vi "Navigation_no s curve may 2.vi"() -> ()   [LabVIEW 2015]
uses:
  <vilib>/myRIO/Instrument Drivers/Onboard IO/PWM/typedefs/PWM Reference.ctl
  <vilib>/myRIO/Common/Instrument Driver Framework/Utilities/typedefs/myRIO Generic Hardware Reference.ctl
  <vilib>/myRIO/Common/Instrument Driver Framework/Utilities/typedefs/Hardware Version Enum.ctl
  <vilib>/myRIO/Common/Instrument Driver Framework/Utilities/typedefs/myRIO v1.0 Reference.ctl
  <vilib>/myRIO/Common/Instrument Driver Framework/Utilities/typedefs/Generic FPGA Reference.ctl
  <vilib>/myRIO/Common/Instrument Driver Framework/myRIO v1.0/PWM/typedefs/PWM Channels Enum.ctl
  <vilib>/myRIO/Instrument Drivers/Onboard IO/PWM/typedefs/PWM Configuration.ctl
  <vilib>/userdefined/High Color/nirio_resource_hc.ctl
  <vilib>/myRIO/Common/Instrument Driver Framework/myRIO v1.0/PWM/vis/myRIO v1.1 Open PWM.vi
  <vilib>/myRIO/Common/Instrument Driver Framework/Utilities/vis/Validate Channels.vi
  <vilib>/myRIO/Common/Instrument Driver Framework/myRIO v1.0/PWM/vis/myRIO v1.0 Reserve PWM.vi
  <vilib>/myRIO/Common/Instrument Driver Framework/myRIO v1.0/PWM/vis/myRIO v1.0 Build MUX Configuration PWM.vi
  <vilib>/myRIO/Common/Instrument Driver Framework/myRIO v1.0/Resource Manager/vis/myRIO v1.0 Reserve Channel List.vi
  <vilib>/myRIO/Common/Instrument Driver Framework/myRIO v1.0/Resource Manager/vis/myRIO v1.0 Create Configuration List.vi
  <vilib>/myRIO/Common/Instrument Driver Framework/myRIO v1.0/Resource Manager/vis/myRIO v1.0 Reserve Channel.vi
  <vilib>/myRIO/Common/Instrument Driver Framework/myRIO v1.0/Resource Manager/vis/myRIO v1.0 Unreserve Channel.vi
  <vilib>/myRIO/Common/Instrument Driver Framework/myRIO v1.0/Resource Manager/vis/myRIO v1.0 Build Mutex Name.vi
  <vilib>/FPGAPlugInAG/myRIO-1900/niLvFpga_Open_myRIO-1900.vi
  <vilib>/rvi/interface/common/dynamic/niFpgaDynamicAddResources.vi
  <vilib>/myRIO/Common/Instrument Driver Framework/Utilities/vis/FPGA Ref Manager.vi
  <vilib>/Utility/error.llb/Error Cluster From Error Code.vi
  <vilib>/myRIO/Common/Instrument Driver Framework/Utilities/vis/Ref Counter.vi
  <vilib>/rvi/errors/niLvFpgaAdjustHostInterfaceError.vi
  <vilib>/Utility/VariantDataType/GetNumericInfo.vi
  <vilib>/myRIO/Common/Instrument Driver Framework/myRIO v1.0/myRIO v1.1 Open.vi
  <vilib>/myRIO/Common/Instrument Driver Framework/Utilities/vis/IO Manager.vi
  <vilib>/myRIO/Common/Instrument Driver Framework/Utilities/vis/Configuration Manager.vi
  <vilib>/myRIO/Common/Instrument Driver Framework/myRIO v1.0/Resource Manager/vis/myRIO v1.0 Configure IO.vi
  <vilib>/myRIO/Common/Instrument Driver Framework/myRIO v1.0/myRIO v1.0 Close.vi
  <vilib>/myRIO/Common/Instrument Driver Framework/myRIO v1.0/PWM/vis/myRIO v1.0 Write PWM.vi
  <vilib>/addons/control/pid/pid.llb/PID (DBL).vi
  <vilib>/rvi/interface/nirviOpenFPGA/nirviOpenFPGA.xnode
  FPGA Bitfiles/NavigationProjec_FPGATarget2_FPGAMainNavigati_PWPHW8gwDxI.lvbitx
  <vilib>/rvi/interface/nirviReadWriteControl/nirviReadWriteControl.xnode
  <vilib>/myRIO/Instrument Drivers/Onboard IO/PWM/vis/myRIO PWM Open.xnode
  <vilib>/myRIO/Instrument Drivers/Onboard IO/PWM/PWM.lvlib
  <vilib>/myRIO/Instrument Drivers/Utilities/Utilities.lvlib
  NiFpgaLv.dll
  <vilib>/rvi/interface/Simulation/niFpgaSimulationCallBeginRW.vi
  <vilib>/addons/control/pid/NI_PID_pid.lvlib
panel:
  out "xstart_return":dbl
  out "goal reached 2":bool=TRUE
  out "percent away from x goal 2":dbl
  out "forward reverse":dbl
  out "big red button":i16
  out "y1ahead":dbl
  out "angle error":dbl
  out "percent away from x goal":dbl
  out "y desired":dbl
  out "slope desired":dbl
  out "orientation theta desired":dbl
  out "current angle":dbl
  out "current y":dbl
  out "current x":dbl
  out "mining angle":dbl
  out "mining y":dbl
  out "mining x":dbl
  out "mining location":dbl=1.0
  out "distance to goal":dbl
  out "loc_y":dbl
  out "loc_x":dbl
  out "loc_theta":dbl
  in  "motor killswitch":bool=TRUE
  in  "set start position":bool
  in  "dumping complete":bool
  in  "digging complete?":bool
  in  "position good?":bool
  in  "state":dbl
  in  "x goal":dbl=9.0
  in  "Encoder Reset":bool
  out "scale":dbl=1.0
  out "reset x y 2":dbl
  out "stop motors":dbl
  out "encoder stop switch":dbl=1.0
  out "left wheels actual pwm":dbl
  out "right wheels actual pwm":dbl
  out "desired pwm right":dbl
  out "desired pwm left":dbl
  out "left setpoint":dbl
  out "right setpoint":dbl
  in  "PID Settings":enum32{"Right PID PWM", "Left PID PWM"}(tab)
  in  "output range right":cluster{"output high":dbl, "output low":dbl}={"output high"=0.13333, "output low"=-0.13333} {"output low" format="%.6f"; "output high" format="%.5f"}
  in  "PID gains right":T1={"proportional gain (Kc)"=0.002, "integral time (Ti, min)"=7e-07, "derivative time (Td, min)"=0.0} {"derivative time (Td, min)" format="%.8f"; "integral time (Ti, min)" format="%.8f"; "proportional gain (Kc)" format="%.8f"}
  out "dt out (s) right":dbl format="%.3f"
  out "PID feedback Right":dbl
  out "Elapsed Time (s) Right":dbl caption="Elapsed Time (s)"
  in  "pid reset right":bool
  in  "output range left":cluster{"output high":dbl, "output low":dbl}={"output high"=0.13333, "output low"=-0.13333} {"output low" format="%.6f"; "output high" format="%.5f"}
  in  "PID gains left":T1={"proportional gain (Kc)"=0.002, "integral time (Ti, min)"=7e-07, "derivative time (Td, min)"=0.0} {"derivative time (Td, min)" format="%.8f"; "integral time (Ti, min)" format="%.8f"; "proportional gain (Kc)" format="%.8f"}
  out "dt out (s) left":dbl format="%.3f"
  out "PID feedback Left":dbl
  out "Elapsed Time (s) Left":dbl caption="Elapsed Time (s)"
  in  "pid reset left":bool
  out "start angle":dbl=1.0
  out "start x":dbl=1.0
  out "start y":dbl
  in  "stuff that i dont want to mess with right now":T2(tab)
  out "RM Linear Velocity (rot/s)":dbl
  out "RR Rot Velocity (rot/s)":dbl
  out "LR Rot Velocity (rot/s)":dbl
  out "LM Rot Velocity (rot/s)":dbl
  out "LF Rot Velocity (rot/s)":dbl
  out "RF Linear Velocity (rot/s)":dbl
  out "Tick Count(mSec) 2":u32 caption="Tick Count(mSec)"
  out "y traveled 2":dbl
  out "x traveled 2":dbl
  out "y position 2":dbl
  out "x position 2":dbl
  out "y dot 2":dbl
  out "distance traveled 2":dbl
  out "psi dot 2":dbl
  out "x dot 2":dbl
  out ".not. x? 2":bool
  out ".not. x? 3":bool
  out "goal reached":bool=TRUE
  out "avg ENC.B":dbl
  out "avg ENC.A":dbl
  out "ENC.B_c.CNTR":i32
  out "ENC.B_b.CNTR":i32
  out "ENC.B_a.CNTR":i32
  out "ENC.A_c.CNTR":i32
  out "ENC.A_b.CNTR":i32
  out "ENC.A_a.CNTR":i32
  out "stage set point parameters":T3(tab)
  in  "x straight 1 end":dbl=2.0
  in  "ypstart straight 1":dbl
  in  "ystart":dbl=1.0
  in  "yend straight 1":dbl=2.0
  in  "ypend straight 1":dbl
  out "a":dbl
  out "b":dbl
  out "c":dbl
  out "d":dbl
  out "x turn end":dbl=7.0
  out "x straight 2 end":dbl=10.0
  in  "mining y 1":dbl=2.0
  in  "mining angle 1":dbl
  in  "mining x 1":dbl=9.0
  in  "mining angle -1":dbl
  in  "mining y -1":dbl=4.0
  in  "mining x -1":dbl=9.0
  out "left pwm":dbl(graph)
  out "right pwm":dbl(graph)
  out "SYS.SELECTA":u8 format="%08b"
  in  "R Min Linear Velocity (ft/s)":dbl=-2.0 format="%#_13g"
  in  "R Max Linear Velocity (ft/s)":dbl=2.0 format="%#_13g"
  in  "L Min Linear Velocity (ft/s)":dbl=-2.0 format="%#_13g"
  in  "L Max Linear Velocity (ft/s)":dbl=2.0 format="%#_13g"
  out "Current Rot Velocity (rot/s)":T4(graph)
  # "Position Information"
  # "move cases along"
  # "end state 0\ngo to state 1"
  # "end state 1\ngo to state 2"
  # "end state 2\ngo to state 3"
  # "end state 3\ngo to state 4"
  # "end state 4\ngo to state 0"
  # "same thing, redundant \nbut can be changed to \nsomething useful later"
  # "this must be true to \ninitialize the routine"
  # "go through the 3\n movement cases"
  # "go through the 3\n movement cases"
  # "Stop Flags \n1=go \n0=stop"
  # "PWM Setpoint"
  # "Initial condtions"
  # "Encoder Values"
  # "Motor Control Parameters"
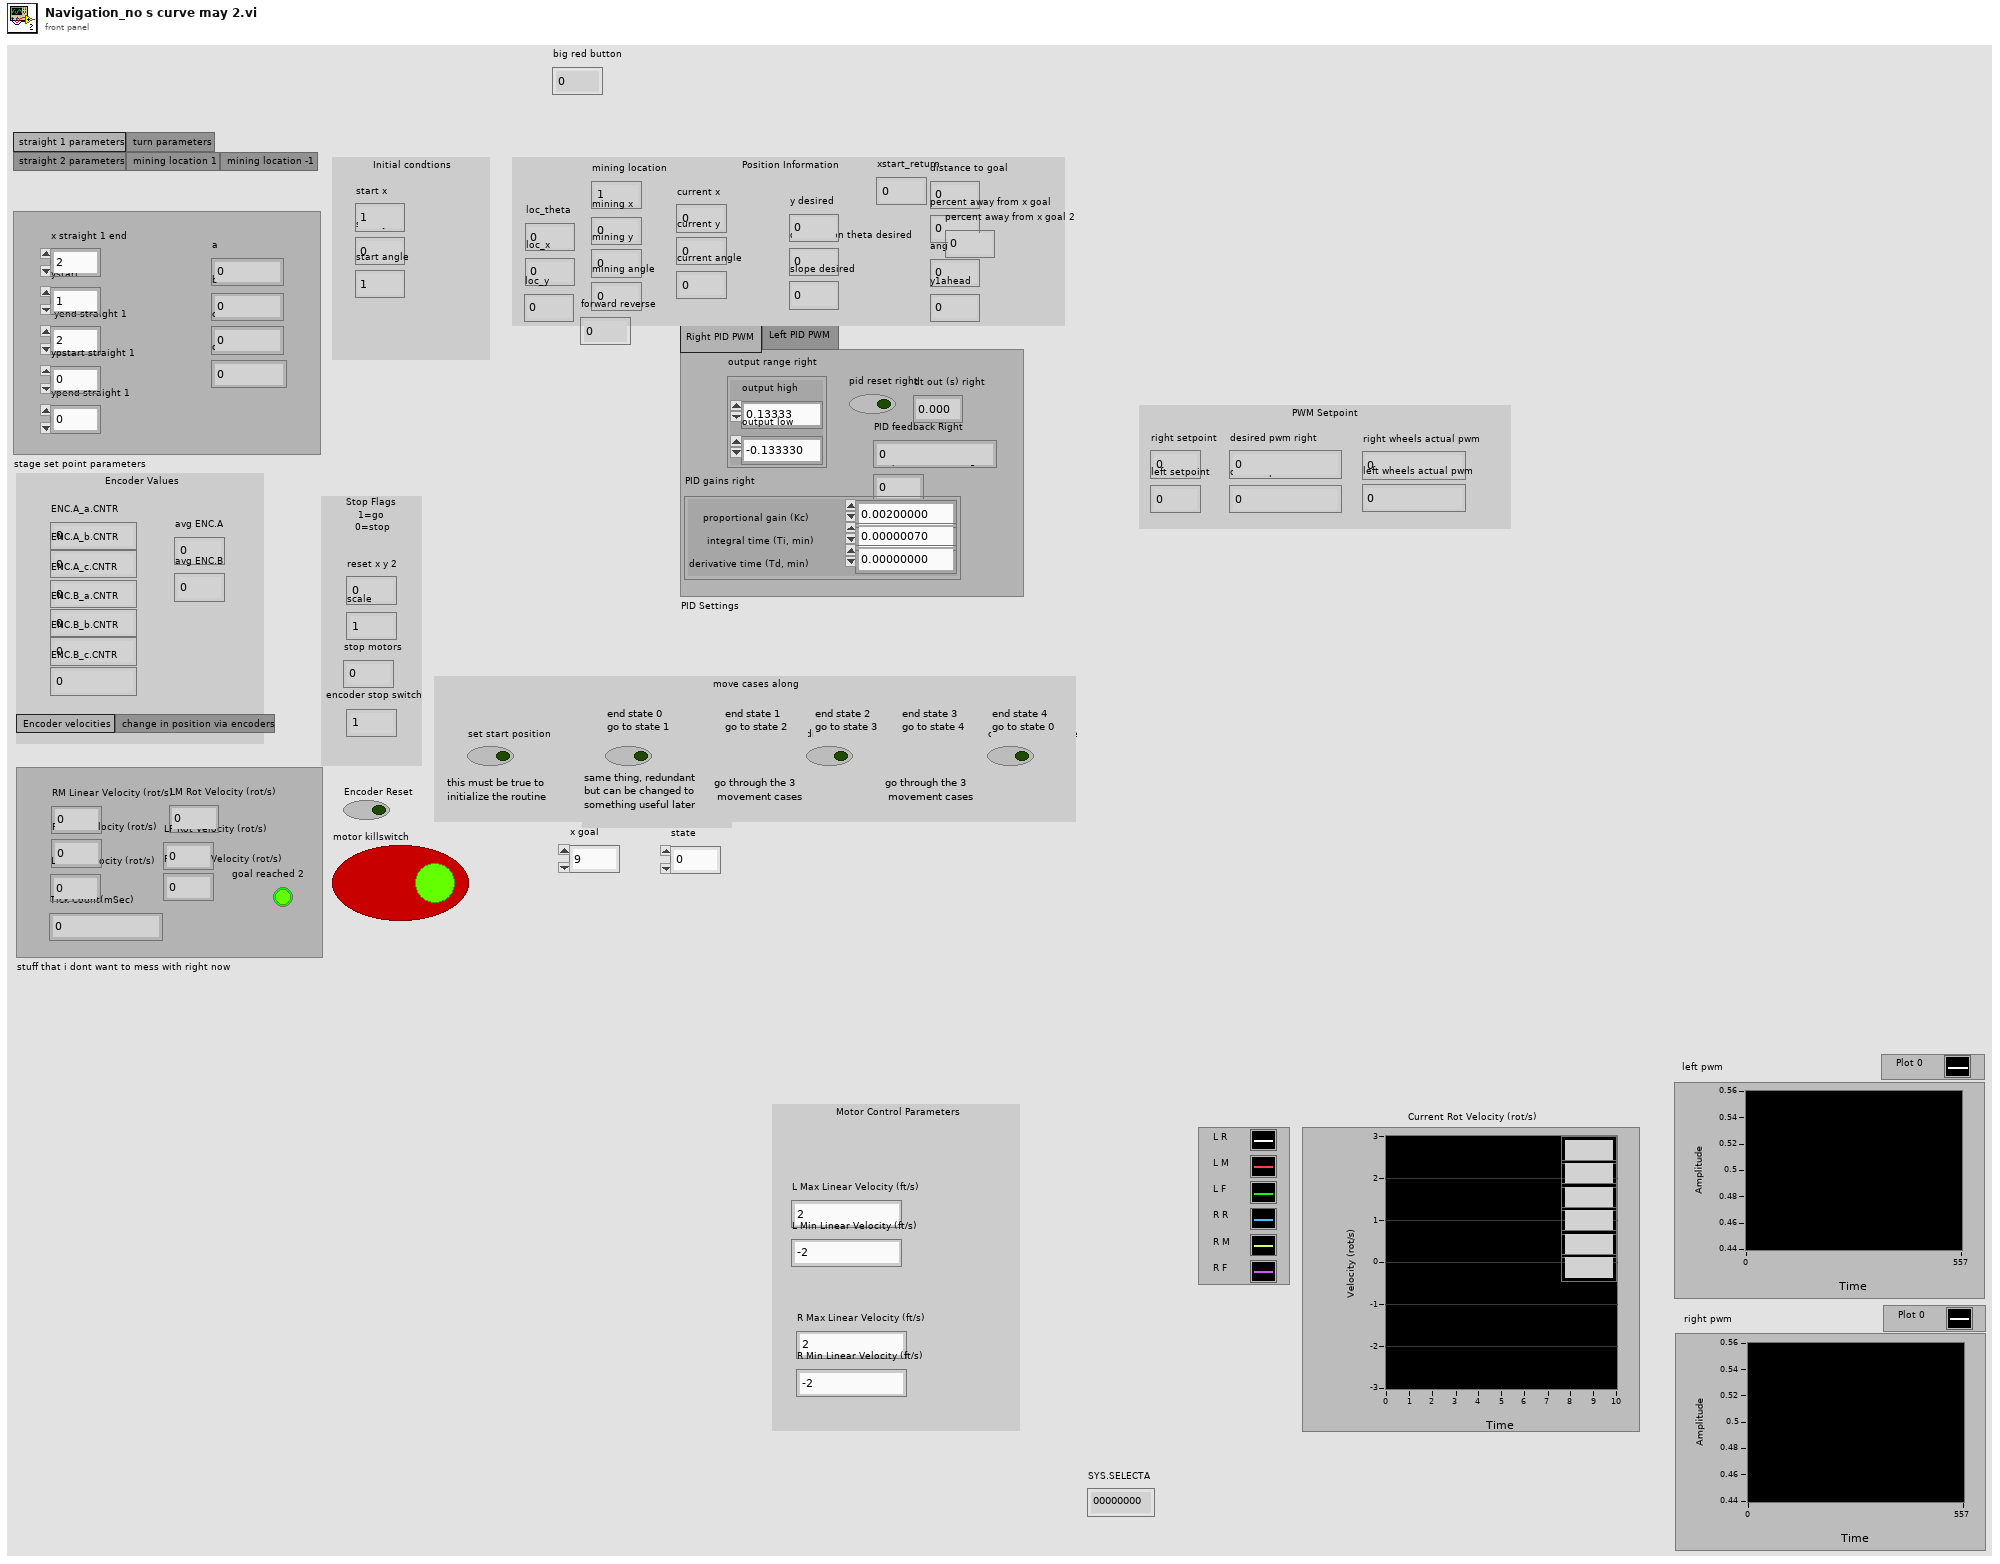
[diagram p1: front panel]
types:
  T1 = cluster{"proportional gain (Kc)":dbl, "integral time (Ti, min)":dbl, "derivative time (Td, min)":dbl}
  T2 = enum32{"Encoder velocities", "change in position via encoders"}
  T3 = enum32{"straight 1 parameters", "turn parameters", "straight 2 parameters", "mining location 1", "mining location -1"}
  T4 = cluster{"Rotational Velocity (RPS)":dbl, "Rotational Velocity (RPS)":dbl, "Rotational Velocity (RPS)":dbl, "Rotational Velocity (RPS)":dbl, "Rotational Velocity (RPS)":dbl, "Rotational Velocity (RPS)":dbl}
  T5 = typedef "nirio_resource_hc.ctl" = tag
  T6 = typedef "Hardware Version Enum.ctl" = enum16{"Unknown", "myRIO-1900", "myRIO-1950", "roboRIO"}
  T7 = typedef "PWM.lvlib/PWM Reference.ctl" = cluster{"myRIO Reference":T8, "PWM Channels Enum":T11, "PWM Configuration":T12}
  T8 = typedef "myRIO Generic Hardware Reference.ctl" = cluster{"myRIO Model":T6, "myRIO Hardware Reference":T9}
  T9 = typedef "myRIO v1.0 Reference.ctl" = cluster{"Generic FPGA Reference":T10, "Allow multiple opens":bool}
  T10 = typedef "Generic FPGA Reference.ctl" = refnum<k20>
  T11 = typedef "PWM Channels Enum.ctl" = enum16{"Not Connected", "C/PWM0", "C/PWM1", "A/PWM0", "A/PWM1", "A/PWM2", "B/PWM0", "B/PWM1", "B/PWM2", "PWM/PWM0", "PWM/PWM1", "PWM/PWM2", "PWM/PWM3", "PWM/PWM4", "PWM/PWM5", "PWM/PWM6", "PWM/PWM7", "PWM/PWM8", "PWM/PWM9"}
  T12 = typedef "PWM.lvlib/PWM Configuration.ctl" = cluster{"Frequency":dbl, "Duty Cycle":dbl}
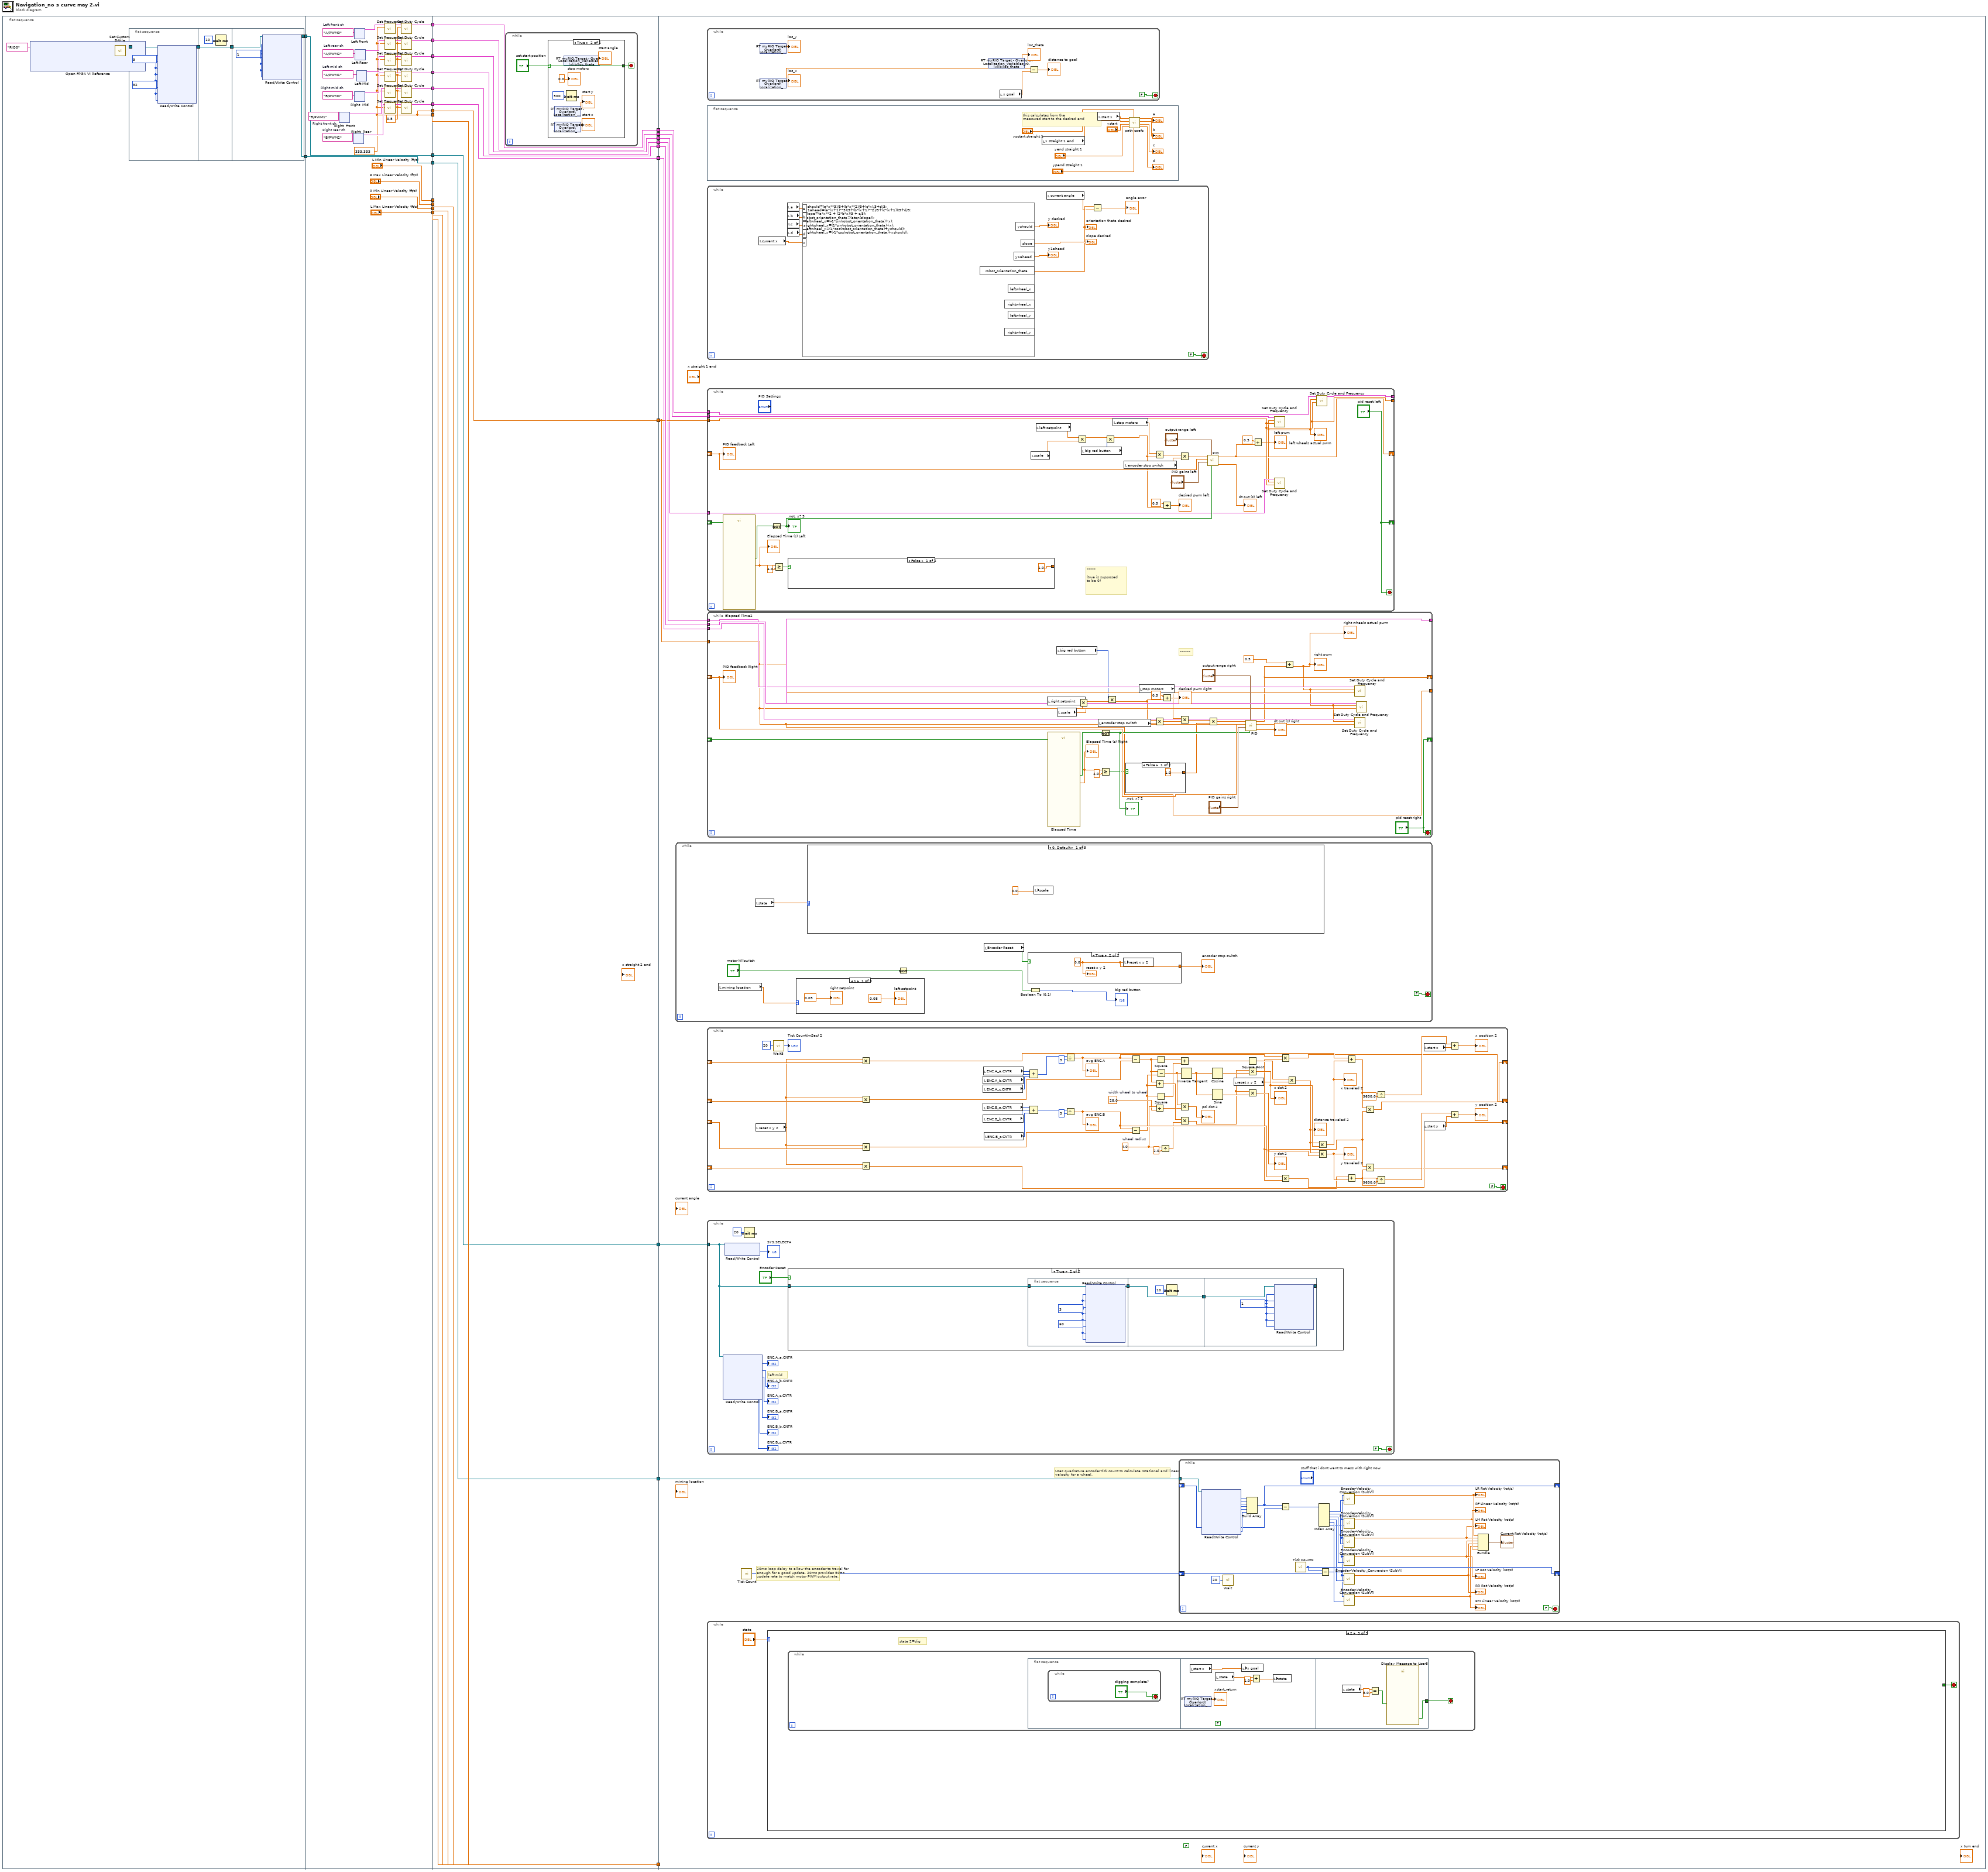
[diagram p0: block diagram]
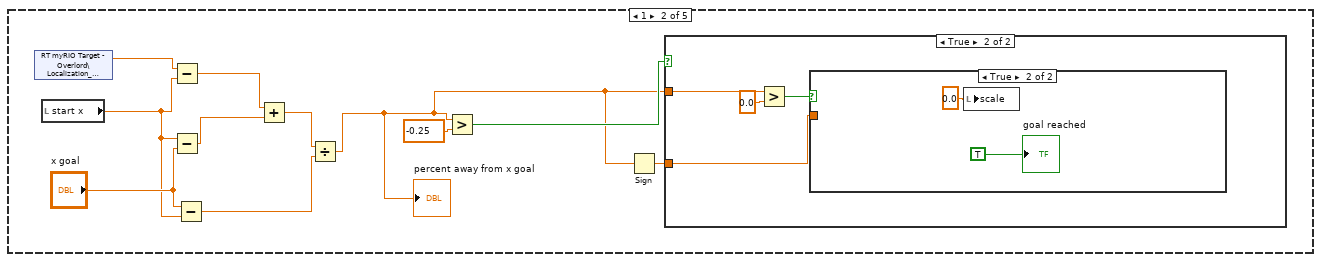
[diagram p3: hidden frame]
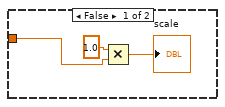
[diagram p4: hidden frame]
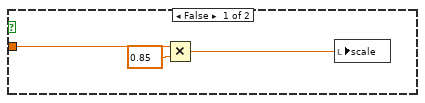
[diagram p5: hidden frame]
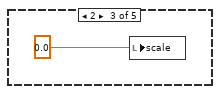
[diagram p6: hidden frame]
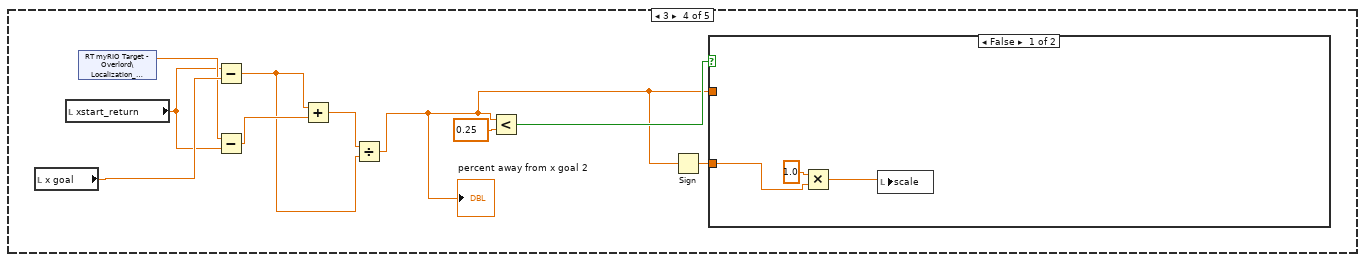
[diagram p7: hidden frame]
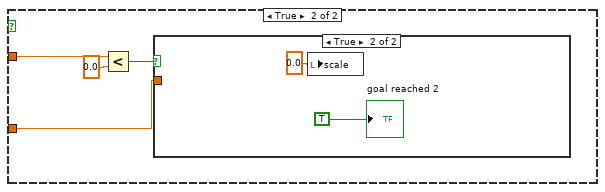
[diagram p8: hidden frame]
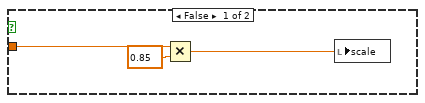
[diagram p9: hidden frame]
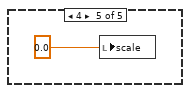
[diagram p10: hidden frame]
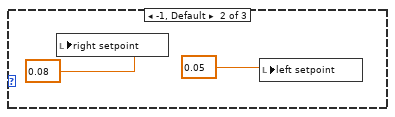
[diagram p11: hidden frame]
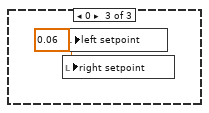
[diagram p12: hidden frame]
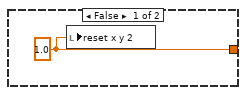
[diagram p13: hidden frame]
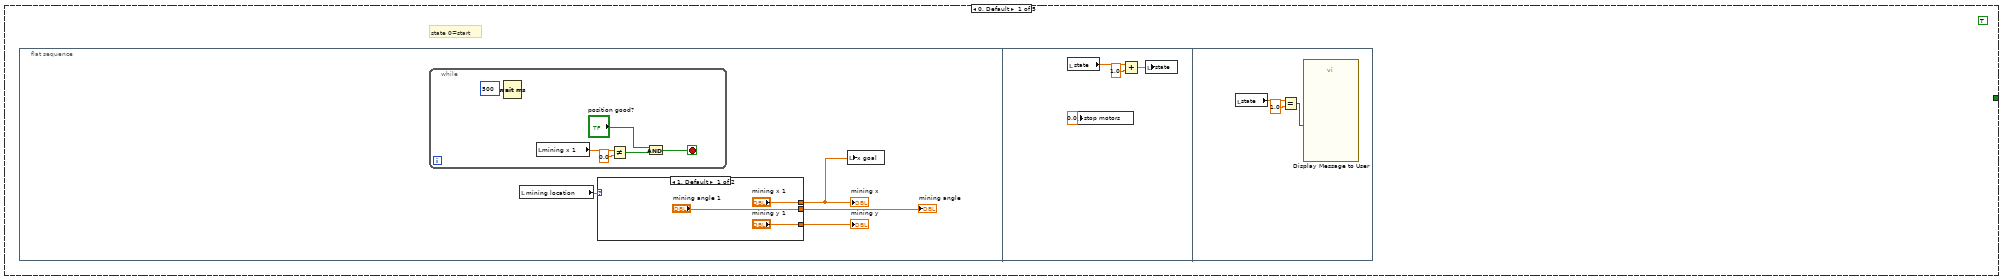
[diagram p14: hidden frame]
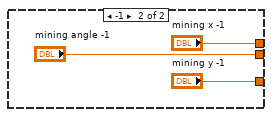
[diagram p15: hidden frame]
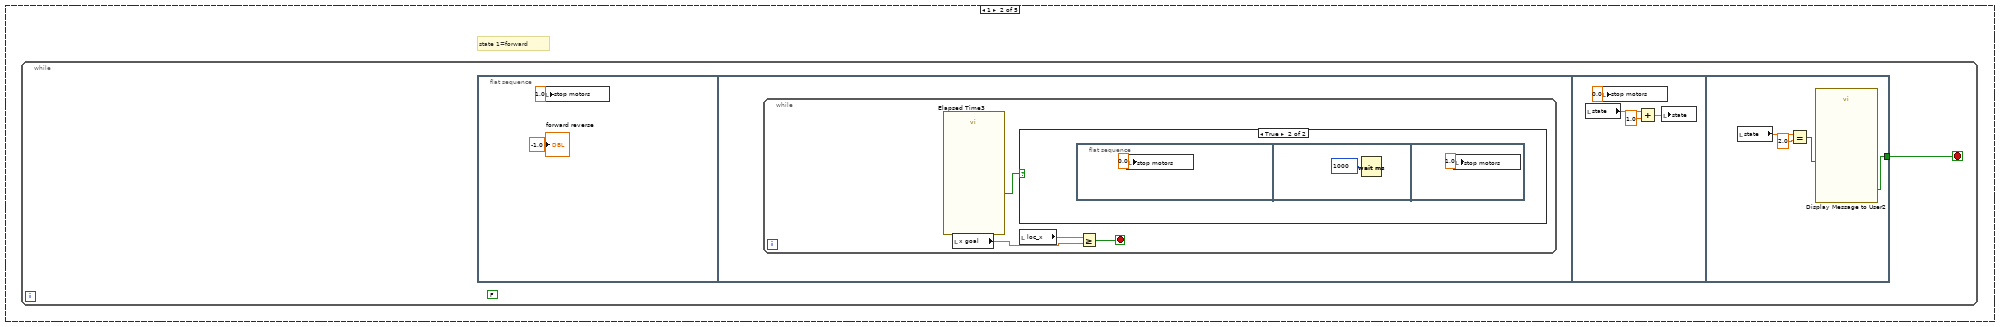
[diagram p16: hidden frame]
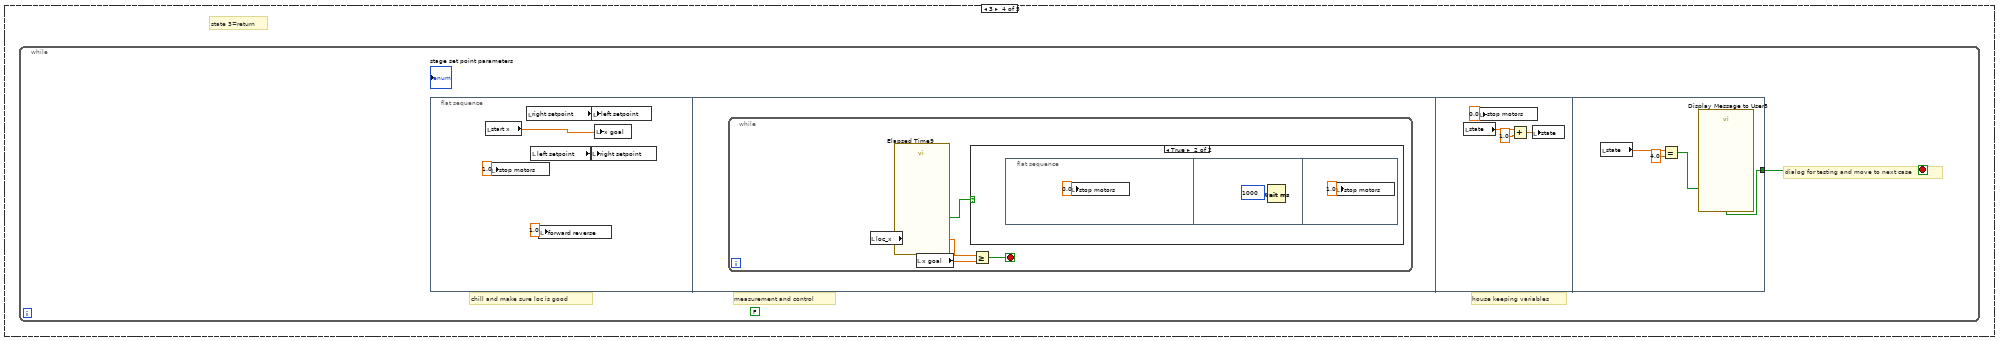
[diagram p18: hidden frame]
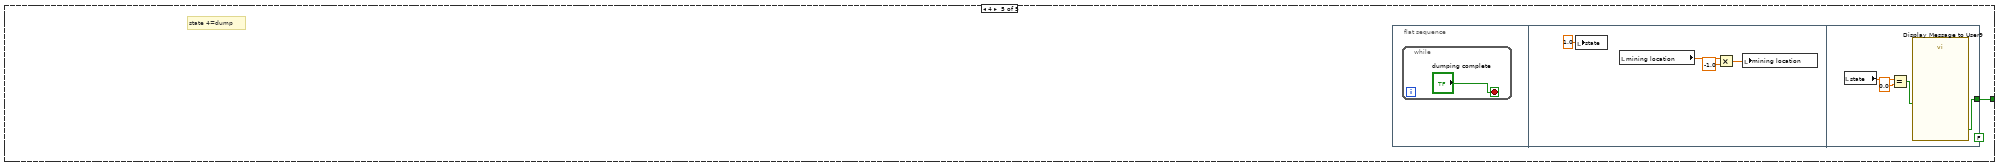
[diagram p20: hidden frame]
diagram:
  n1 = flat-sequence {
    tunnel: [w33] -> w30
    tunnel: [w33] -> w29
    tunnel: [w46] -> w28
    tunnel: [w61] -> w26
    tunnel: [w57] -> w24
    tunnel: [w56] -> w22
    tunnel: [w55] -> w20
    tunnel: [w54] -> w18
    tunnel: [w53] -> w16
    tunnel: ["L Max Linear Velocity (ft/s)"] -> w14
    tunnel: ["L Min Linear Velocity (ft/s)"] -> w12
    tunnel: ["R Max Linear Velocity (ft/s)"] -> w10
    tunnel: ["R Min Linear Velocity (ft/s)"] -> w8
    tunnel: [w48] -> w6
    tunnel: w30 -> [w47]
    tunnel: [w47] -> w4
    tunnel: w29 -> [w48]
    tunnel: [w46] -> w2
    tunnel: w28 -> [w187]
    tunnel: [w187] -> w27
    tunnel: w26 -> [w186]
    tunnel: [w186] -> w25
    tunnel: w24 -> [w185]
    tunnel: [w185] -> w23
    tunnel: w22 -> [w184]
    tunnel: [w184] -> w21
    tunnel: w20 -> [w183]
    tunnel: [w183] -> w19
    tunnel: w18 -> [w182]
    tunnel: [w182] -> w17
    tunnel: w16 -> [w181]
    tunnel: [w181] -> w15
    tunnel: w14 -> [w180]
    tunnel: [w180] -> w13
    tunnel: w12 -> [w179]
    tunnel: [w179] -> w11
    tunnel: w10 -> [w178]
    tunnel: [w178] -> w9
    tunnel: w8 -> [w177]
    tunnel: [w177] -> w7
    tunnel: w6 -> [w176]
    tunnel: [w176] -> w5
    tunnel: w4 -> [w175]
    tunnel: [w175] -> w3
    tunnel: w2 -> [w174]
    tunnel: [w174] -> w1
    tunnel: w27 -> [_]
    tunnel: w25 -> [w196]
    tunnel: w23 -> [w202]
    tunnel: w21 -> [w199]
    tunnel: w19 -> [w198]
    tunnel: w17 -> [w197]
    tunnel: w15 -> [w201]
    tunnel: w13 -> [_]
    tunnel: w11 -> [_]
    tunnel: w9 -> [_]
    tunnel: w7 -> [_]
    tunnel: w5 -> [w204]
    tunnel: w3 -> [w203]
    tunnel: w1 -> [w200]
    frame #0 {
      n2 = xnode "Open FPGA VI Reference"("resource name"=tag "RIO0") -> ("FPGA VI Reference Out"=w32:refnum<k20>)  [unwired: 1 in, 1 out]
      n3 = call <vilib>:"Set Custom Bitfile.vi"("Custom FPGA Reference In"=w32) -> ("Custom FPGA Reference Out"=w34:refnum<k20>)  [unwired: 9 in, 1 out]
      n4 = flat-sequence {
        tunnel: w34 -> [w39]
        tunnel: [w37] -> w36
        tunnel: w36 -> [w41]
        tunnel: [w41] -> w35
        tunnel: w35 -> [w44]
        tunnel: [w43] -> w33
        frame #0 {
          w38 = u8 32 ("SYS.SELECTA")
          w40 = u8 3 ("ENC.B_c.CNFG")
          n5 = xnode "Read/Write Control"("FPGA VI Reference In"=w39, "ENC.A_a.CNFG"=w40, "ENC.A_b.CNFG"=w40, "ENC.A_c.CNFG"=w40, "ENC.B_a.CNFG"=w40, "ENC.B_b.CNFG"=w40, "ENC.B_c.CNFG"=w40, "SYS.SELECTA"=w38, "SYS.SELECTB"=w38) -> ("FPGA VI Reference Out"=w37:refnum<k20>)  [unwired: 1 in, 1 out]
        }
        frame #1 {
          n6 = Wait (ms)(milliseconds to wait=u32 10) -> ()  [unwired: 1 out]
        }
        frame #2 {
          w45 = u8 1 ("ENC.B_c.CNFG")
          n7 = xnode "Read/Write Control"("FPGA VI Reference In"=w44, "ENC.A_a.CNFG"=w45, "ENC.A_b.CNFG"=w45, "ENC.A_c.CNFG"=w45, "ENC.B_a.CNFG"=w45, "ENC.B_b.CNFG"=w45, "ENC.B_c.CNFG"=w45) -> ("FPGA VI Reference Out"=w43:refnum<k20>)  [unwired: 1 in, 1 out]
        }
      }
    }
    frame #1 {
      w58 = 0.5 ("Duty Cycle")
      w46 = 333.333 ("Frequency [Hz]")
      w72 = tag "B/PWM2"  # Right rear ch
      w73 = tag "B/PWM0"  # Right mid ch
      w74 = tag "B/PWM1"  # Right front ch
      w75 = tag "A/PWM2"  # Left rear ch
      w76 = tag "A/PWM1"  # Left mid ch
      w77 = tag "A/PWM0"  # Left front ch
      n8 = xnode "Right  Front"("Channel Name"=w74) -> ("PWM Ref Out"=w68:T7)  [unwired: 2 in, 1 out]
      n9 = xnode "Right  Rear"("Channel Name"=w72) -> ("PWM Ref Out"=w66:T7)  [unwired: 2 in, 1 out]
      n10 = xnode "Left Front"("Channel Name"=w77) -> ("PWM Ref Out"=w71:T7)  [unwired: 2 in, 1 out]
      n11 = xnode "Right  Mid"("Channel Name"=w73) -> ("PWM Ref Out"=w67:T7)  [unwired: 2 in, 1 out]
      n12 = xnode "Left Rear"("Channel Name"=w75) -> ("PWM Ref Out"=w69:T7)  [unwired: 2 in, 1 out]
      n13 = xnode "Left Mid"("Channel Name"=w76) -> ("PWM Ref Out"=w70:T7)  [unwired: 2 in, 1 out]
      n14 = call <vilib>:"Set Frequency.vi"("Frequency [Hz]"=w46, "PWM Ref In"=w71) -> ("PWM Ref Out"=w65:T7)  [unwired: 7 in, 1 out]
      n15 = call <vilib>:"Set Frequency.vi"("Frequency [Hz]"=w46, "PWM Ref In"=w69) -> ("PWM Ref Out"=w60:T7)  [unwired: 7 in, 1 out]
      n16 = call <vilib>:"Set Frequency.vi"("Frequency [Hz]"=w46, "PWM Ref In"=w70) -> ("PWM Ref Out"=w59:T7)  [unwired: 7 in, 1 out]
      n17 = call <vilib>:"Set Frequency.vi"("Frequency [Hz]"=w46, "PWM Ref In"=w67) -> ("PWM Ref Out"=w63:T7)  [unwired: 7 in, 1 out]
      n18 = call <vilib>:"Set Frequency.vi"("Frequency [Hz]"=w46, "PWM Ref In"=w68) -> ("PWM Ref Out"=w62:T7)  [unwired: 7 in, 1 out]
      n19 = call <vilib>:"Set Frequency.vi"("Frequency [Hz]"=w46, "PWM Ref In"=w66) -> ("PWM Ref Out"=w64:T7)  [unwired: 7 in, 1 out]
      n20 = call <vilib>:"Set Duty Cycle.vi"("Duty Cycle"=w58, "PWM Ref In"=w65) -> ("PWM Ref Out"=w53:T7)  [unwired: 7 in, 1 out]
      n21 = call <vilib>:"Set Duty Cycle.vi"("Duty Cycle"=w58, "PWM Ref In"=w60) -> ("PWM Ref Out"=w61:T7)  [unwired: 7 in, 1 out]
      n22 = call <vilib>:"Set Duty Cycle.vi"("Duty Cycle"=w58, "PWM Ref In"=w59) -> ("PWM Ref Out"=w54:T7)  [unwired: 7 in, 1 out]
      n23 = call <vilib>:"Set Duty Cycle.vi"("Duty Cycle"=w58, "PWM Ref In"=w63) -> ("PWM Ref Out"=w56:T7)  [unwired: 7 in, 1 out]
      n24 = call <vilib>:"Set Duty Cycle.vi"("Duty Cycle"=w58, "PWM Ref In"=w62) -> ("PWM Ref Out"=w57:T7)  [unwired: 7 in, 1 out]
      n25 = call <vilib>:"Set Duty Cycle.vi"("Duty Cycle"=w58, "PWM Ref In"=w64) -> ("PWM Ref Out"=w55:T7)  [unwired: 7 in, 1 out]
    }
    frame #2 {
      n26 = while {
        stop <- w188 stop-if-true
        n27 = case shown="True" "set start position" {
          selector: "set start position" -> [_ w195]
          tunnel: [_ w195] -> w188
          frame False {
          }
          frame True {
            n28 = shared-variable "RT myRIO Target - Overlord\\Localization_Variables_r0.lvlib\\loc_y"() -> (→"start y":dbl)  [unwired: 1 in, 1 out]
            n29 = shared-variable "RT myRIO Target - Overlord\\Localization_Variables_r0.lvlib\\loc_x"() -> (→"start x":dbl)  [unwired: 1 in, 1 out]
            n30 = shared-variable "RT myRIO Target - Overlord\\Localization_Variables_r0.lvlib\\loc_theta"() -> (→"start angle":dbl)  [unwired: 1 in, 1 out]
            n31 = Wait (ms)(milliseconds to wait=u32 500) -> ()  [unwired: 1 out]
            "stop motors" <- 0.0 ("stop motors")
          }
        }
      }
    }
    frame #3 {
      (unwired) FALSE
      # "Uses quadrature encoder tick count to calculate rotational and linear velocity for a wheel."
      # "20ms loop delay to allow the encoder to travel far enough for a good update. 20ms provides 50Hz update rate to match motor PWM output rate."
      n32 = while {
        stop <- FALSE stop-if-true
        n33 = local read "mining location"() -> (w207:dbl)
        n34 = local read "state"() -> (w206:dbl)
        n35 = case shown="1" w207 {
          frame 1 {
            "right setpoint" <- 0.05
            "left setpoint" <- 0.08
          }
          frame -1, Default {
            n36 = local write "right setpoint"(0.08) -> ()
            n37 = local write "left setpoint"(0.05) -> ()
          }
          frame 0 {
            w266 = 0.06 ("left setpoint")
            n38 = local write "right setpoint"(w266) -> ()
            n39 = local write "left setpoint"(w266) -> ()
          }
        }
        n40 = case shown="0, Default" w206 {
          frame 0, Default {
            n41 = local write "scale"(0.0) -> ()
          }
          frame 1 {
            n42 = shared-variable "RT myRIO Target - Overlord\\Localization_Variables_r0.lvlib\\loc_x"() -> (w224:dbl)  [unwired: 1 in, 1 out]
            n43 = local read "start x"() -> (w219:dbl)
            n44 = Subtract(x=w224, y=w219) -> (x-y=w223:dbl)
            n45 = Subtract(x=w219, y="x goal") -> (x-y=w222:dbl)
            n46 = Subtract(x="x goal", y=w219) -> (x-y=w218:dbl)
            n47 = Add(x=w223, y=w222) -> (x+y=w221:dbl)
            n48 = Divide(x=w221, y=w218) -> (x/y=w216:dbl)
            "percent away from x goal" <- w216
            n49 = Greater?(x=w216, y=-0.25) -> (0:w217:bool)
            n50 = Sign(1:w216) -> (0:w215:dbl)
            n51 = case shown="True" w217 {
              tunnel: w216 -> [_ w232]
              tunnel: w215 -> [w226 w229]
              frame False {
                n52 = Multiply(x=1.0, y=w226) -> (x*y=→"scale":dbl)
              }
              frame True {
                n53 = Greater?(x=w232, y=0.0) -> (0:w230:bool)
                n54 = case shown="True" w230 {
                  tunnel: w229 -> [w235 _]
                  frame False {
                    n55 = Multiply(x=w235, y=0.85) -> (x*y=w233:dbl)
                    n56 = local write "scale"(w233) -> ()
                  }
                  frame True {
                    n57 = local write "scale"(0.0) -> ()
                    "goal reached" <- TRUE
                  }
                }
              }
            }
          }
          frame 2 {
            n58 = local write "scale"(0.0) -> ()
          }
          frame 3 {
            n59 = local read "x goal"() -> (w242:dbl)
            n60 = local read "xstart_return"() -> (w240:dbl)
            n61 = shared-variable "RT myRIO Target - Overlord\\Localization_Variables_r0.lvlib\\loc_x"() -> (w241:dbl)  [unwired: 1 in, 1 out]
            n62 = Subtract(x=w240, y=w242) -> (x-y=w239:dbl)
            n63 = Subtract(x=w241, y=w240) -> (x-y=w247:dbl)
            n64 = Add(x=w239, y=w247) -> (x+y=w246:dbl)
            n65 = Divide(x=w246, y=w239) -> (x/y=w244:dbl)
            "percent away from x goal 2" <- w244
            n66 = Less?(x=w244, y=0.25) -> (x < y?=w245:bool)
            n67 = Sign(1:w244) -> (0:w243:dbl)
            n68 = case shown="False" w245 {
              tunnel: w244 -> [_ w255]
              tunnel: w243 -> [w250 w252]
              frame False {
                n69 = Multiply(x=1.0, y=w250) -> (x*y=w249:dbl)
                n70 = local write "scale"(w249) -> ()
              }
              frame True {
                n71 = Less?(x=w255, y=0.0) -> (x < y?=w253:bool)
                n72 = case shown="True" w253 {
                  tunnel: w252 -> [w258 _]
                  frame False {
                    n73 = Multiply(x=w258, y=0.85) -> (x*y=w256:dbl)
                    n74 = local write "scale"(w256) -> ()
                  }
                  frame True {
                    n75 = local write "scale"(0.0) -> ()
                    "goal reached 2" <- TRUE
                  }
                }
              }
            }
          }
          frame 4 {
            n76 = local write "scale"(0.0) -> ()
          }
        }
        n77 = Not(x="motor killswitch") -> (.not. x?=w211:bool)
        n78 = local read "Encoder Reset"() -> (w213:bool)
        n79 = case shown="True" w213 {
          tunnel: [w267 w268] -> w212
          frame False {
            w267 = 1.0
            n80 = local write "reset x y 2"(w267) -> ()
          }
          frame True {
            w268 = 0.0
            n81 = local write "reset x y 2"(w268) -> ()
            "reset x y 2" <- w268
          }
        }
        "encoder stop switch" <- w212
        n82 = Boolean To (0,1)(Boolean=w211) -> (0, 1=→"big red button":i16)
      }
      n83 = while {
        stop <- FALSE stop-if-true
        n84 = shared-variable "RT myRIO Target - Overlord\\Localization_Variables_r0.lvlib\\loc_y"() -> (→"loc_y":dbl)  [unwired: 1 in, 1 out]
        n85 = shared-variable "RT myRIO Target - Overlord\\Localization_Variables_r0.lvlib\\loc_x"() -> (w379:dbl)  [unwired: 1 in, 1 out]
        "loc_x" <- w379
        n86 = shared-variable "RT myRIO Target - Overlord\\Localization_Variables_r0.lvlib\\loc_theta"() -> (→"loc_theta":dbl)  [unwired: 1 in, 1 out]
        n87 = local read "x goal"() -> (w378:dbl)
        n88 = Subtract(x=w379, y=w378) -> (x-y=→"distance to goal":dbl)
      }
      n89 = flat-sequence {
        frame #0 {
          # "this calculates from the \nmeasured start to the desired end"
          n90 = local read "x straight 1 end"() -> (w281:dbl)
          n91 = local read "start x"() -> (w282:dbl)
          n92 = call "path coefs.vi"("ypend"="ypend straight 1", "ypstart"="ypstart straight 1", "yend"="yend straight 1", "ystart"="ystart", "xend"=w281, "xstart"=w282) -> ("d"=→"d":dbl, "c"=→"c":dbl, "b"=→"b":dbl, "a"=→"a":dbl)  [unwired: 2 in]
        }
      }
      n93 = while {
        stop <- FALSE stop-if-true
        n94 = local read "current x"() -> (w275:dbl)
        n95 = local read "a"() -> (w279:dbl)
        n96 = local read "b"() -> (w278:dbl)
        n97 = local read "d"() -> (w276:dbl)
        n98 = local read "c"() -> (w277:dbl)
        n99 = formula code="yshould=(a*x**3)/3+(b*x**2)/3+(c*x)/3+d/3;\ny1ahead=(a*(x+1)**3)/3+(b*(x+1)**2)/3+(c*(x+1))/3+d/3;\nslope=(a*x**2 + (2*b*x)/3 + c/3);\nrobot_orientation_theta=(atan(slope));\nleftwheel_x=(-1*sin(robot_orientation_theta)+x);\nrightwheel_x=(1*sin(robot_orientation_theta)+x);\nleftwheel_y=(1*cos(robot_orientation_theta)+yshould);\nrightwheel_y=(-1*cos(robot_orientation_theta)+yshould);"("a"=w279, "b"=w278, "c"=w277, "d"=w276, "x"=w275) -> ("yshould"=→"y desired":dbl, "slope"=→"slope desired":dbl, "robot_orientation_theta"=w272:dbl, "y1ahead"=→"y1ahead":dbl)  [unwired: 4 out]
        "orientation theta desired" <- w272
        n100 = local read "current angle"() -> (w271:dbl)
        n101 = Subtract(x=w272, y=w271) -> (x-y=→"angle error":dbl)
      }
      n102 = while {
        tunnel: w201 -> [w410]
        tunnel: [w411] -> _
        tunnel: w200 -> [w398]
        shift-right: [w397] -> _
        shift-left: _ -> [w406]
        shift-right: ["pid reset left"] -> _
        shift-left: _ -> [w392]
        tunnel: [w398] -> _
        tunnel: w197 -> [w400]
        tunnel: w196 -> [w399]
        stop <- "pid reset left" stop-if-true
        # "*****\n\n(true is supposed\nto be 0)"
        n103 = call "Elapsed Time2"("Reset"=w392) -> ("Elapsed Time (s)"=w391:dbl, "Time has Elapsed"=w393:bool)  [unwired: 11 in, 6 out]
        "Elapsed Time (s) Left" <- w391
        n104 = Not(x=w393) -> (.not. x?=w405:bool)
        ".not. x? 3" <- w405
        n105 = Greater Or Equal?(x=w391, y=4.0) -> (x >= y?=w389:bool)
        n106 = case shown="False" w389 {
          tunnel: [1.0 1.0] -> _
          frame False {
          }
          frame True {
          }
        }
        n107 = local read "scale"() -> (w383:dbl)
        n108 = local read "left setpoint"() -> (w384:dbl)
        n109 = Multiply(x=w384, y=w383) -> (x*y=w396:dbl)
        n110 = local read "big red button"() -> (w385:i16)
        n111 = Multiply(x=w396, y=w385) -> (x*y=w382:dbl)
        n112 = local read "stop motors"() -> (w401:dbl)
        n113 = local read "encoder stop switch"() -> (w394:dbl)
        n114 = Multiply(x=w401, y=w382) -> (x*y=w395:dbl)
        n115 = Add(x=0.5, y=w382) -> (x+y=→"desired pwm left":dbl)
        n116 = Multiply(x=w395, y=w394) -> (x*y=w386:dbl)
        n117 = call-poly <vilib>:"PID.vi"("reinitialize? (F)"=w405, "output range"="output range left", "PID gains"="PID gains left", "process variable"=w406, "setpoint"=w386) -> ("dt out (s)"=→"dt out (s) left":dbl, "output"=w397:dbl)  [unwired: 5 in]
        n118 = Add(x=0.5, y=w397) -> (x+y=w387:dbl)
        "left wheels actual pwm" <- w387
        "left pwm" <- w387
        n119 = call <vilib>:"Set Duty Cycle and Frequency.vi"("Frequency [Hz]"=w398, "Duty Cycle"=w387, "PWM Ref In"=w399) -> ()  [unwired: 6 in, 2 out]
        n120 = call <vilib>:"Set Duty Cycle and Frequency.vi"("Frequency [Hz]"=w398, "Duty Cycle"=w387, "PWM Ref In"=w400) -> ()  [unwired: 6 in, 2 out]
        n121 = call <vilib>:"Set Duty Cycle and Frequency.vi"("Frequency [Hz]"=w398, "Duty Cycle"=w387, "PWM Ref In"=w410) -> ("PWM Ref Out"=w411:T7)  [unwired: 6 in, 1 out]
        "PID feedback Left" <- w406
      }
      n122 = while {
        tunnel: w202 -> [w506]
        tunnel: [w507] -> _
        tunnel: [w495] -> _
        shift-right: [w494] -> _
        shift-left: _ -> [w502]
        shift-right: ["pid reset right"] -> _
        shift-left: _ -> [w489]
        tunnel: w200 -> [w495]
        tunnel: w199 -> [w497]
        tunnel: w198 -> [w496]
        stop <- "pid reset right" stop-if-true
        # "******"
        n123 = local read "right setpoint"() -> (w478:dbl)
        n124 = call "Elapsed Time"("Reset"=w489) -> ("Elapsed Time (s)"=w488:dbl, "Time has Elapsed"=w486:bool)  [unwired: 11 in, 6 out]
        "Elapsed Time (s) Right" <- w488
        n125 = local read "big red button"() -> (w479:i16)
        n126 = local read "scale"() -> (w477:dbl)
        n127 = Multiply(x=w478, y=w477) -> (x*y=w482:dbl)
        n128 = local read "encoder stop switch"() -> (w492:dbl)
        n129 = Not(x=w486) -> (.not. x?=w501:bool)
        ".not. x? 2" <- w501
        n130 = Greater Or Equal?(x=w488, y=4.0) -> (x >= y?=w485:bool)
        n131 = Multiply(x=w479, y=w482) -> (x*y=w476:dbl)
        n132 = case shown="False" w485 {
          tunnel: [1.0 1.0] -> w490
          frame False {
          }
          frame True {
          }
        }
        n133 = local read "stop motors"() -> (w483:dbl)
        n134 = Multiply(x=w476, y=w492) -> (x*y=w493:dbl)
        n135 = Add(x=0.5, y=w476) -> (x+y=→"desired pwm right":dbl)
        n136 = Multiply(x=w483, y=w493) -> (x*y=w484:dbl)
        n137 = Multiply(x=w484, y=w490) -> (x*y=w491:dbl)
        n138 = call-poly <vilib>:"PID.vi"("reinitialize? (F)"=w501, "output range"="output range right", "PID gains"="PID gains right", "process variable"=w502, "setpoint"=w491) -> ("dt out (s)"=→"dt out (s) right":dbl, "output"=w494:dbl)  [unwired: 5 in]
        n139 = Add(x=0.5, y=w494) -> (x+y=w480:dbl)
        "right wheels actual pwm" <- w480
        "right pwm" <- w480
        n140 = call <vilib>:"Set Duty Cycle and Frequency.vi"("Frequency [Hz]"=w495, "Duty Cycle"=w480, "PWM Ref In"=w497) -> ()  [unwired: 6 in, 2 out]
        n141 = call <vilib>:"Set Duty Cycle and Frequency.vi"("Frequency [Hz]"=w495, "Duty Cycle"=w480, "PWM Ref In"=w496) -> ()  [unwired: 6 in, 2 out]
        n142 = call <vilib>:"Set Duty Cycle and Frequency.vi"("Frequency [Hz]"=w495, "Duty Cycle"=w480, "PWM Ref In"=w506) -> ("PWM Ref Out"=w507:T7)  [unwired: 6 in, 1 out]
        "PID feedback Right" <- w502
      }
      n143 = while {
        shift-right: [w424] -> _
        shift-left: _ -> [w462]
        shift-right: [w421] -> _
        shift-left: _ -> [w461]
        shift-right: [w423] -> _
        shift-left: _ -> [w436]
        shift-right: [w422] -> _
        shift-left: _ -> [w435]
        stop <- FALSE stop-if-true
        w457 = 28.0  # width wheel to wheel
        w458 = 4.0  # wheel radius
        n144 = local read "reset x y 2"() -> (w420:dbl)
        n145 = call "Wait3"("Count(mSec)"=u32 20) -> ("Tick Count(mSec)"=→"Tick Count(mSec) 2":u32)
        n146 = Multiply(x=w420, y=w435) -> (x*y=w426:dbl)
        n147 = Multiply(x=w420, y=w462) -> (x*y=w428:dbl)
        n148 = Multiply(x=w420, y=w461) -> (x*y=w425:dbl)
        n149 = Multiply(x=w420, y=w436) -> (x*y=w427:dbl)
        n150 = local read "ENC.A_b.CNTR"() -> (w469:i32)
        n151 = local read "ENC.A_c.CNTR"() -> (w468:i32)
        n152 = local read "ENC.B_a.CNTR"() -> (w467:i32)
        n153 = local read "ENC.B_b.CNTR"() -> (w466:i32)
        n154 = local read "ENC.A_a.CNTR"() -> (w470:i32)
        n155 = local read "ENC.B_c.CNTR"() -> (w465:i32)
        n156 = Compound Arithmetic op=ADD(w470, w469, w468) -> (w474:i32)
        n157 = Compound Arithmetic op=ADD(w467, w466, w465) -> (w473:i32)
        n158 = Divide(x=w474, y=3) -> (x/y=w463:dbl)
        "avg ENC.A" <- w463
        n159 = Divide(x=w473, y=3) -> (x/y=w460:dbl)
        "avg ENC.B" <- w460
        n160 = Subtract(x=w463, y=w428) -> (x-y=w451:dbl)
        n161 = Subtract(x=w460, y=w425) -> (x-y=w450:dbl)
        n162 = Add(x=w451, y=w450) -> (x+y=w455:dbl)
        n163 = Divide(x=w458, y=w457) -> (x/y=w453:dbl)
        n164 = Square(x=w451) -> (x^2=w448:dbl)
        n165 = Square(x=w450) -> (x^2=w449:dbl)
        n166 = Subtract(x=w451, y=w450) -> (x-y=w454:dbl)
        n167 = Divide(x=w458, y=2.0) -> (x/y=w456:dbl)
        n168 = Add(x=w448, y=w449) -> (x+y=w447:dbl)
        n169 = Multiply(x=w454, y=w453) -> (x*y=→"psi dot 2":dbl)
        n170 = Multiply(x=w455, y=w456) -> (x*y=w444:dbl)
        n171 = Inverse Tangent(1:w454) -> (0:w452:dbl)
        n172 = Cosine(x=w452) -> (cos(x)=w445:dbl)
        n173 = Sine(x=w452) -> (sin(x)=w446:dbl)
        n174 = local read "reset x y 2"() -> (w418:dbl)
        n175 = Square Root(x=w447) -> (sqrt(x)=w441:dbl)
        n176 = Multiply(x=w444, y=w445) -> (x*y=w442:dbl)
        "x dot 2" <- w442
        n177 = Multiply(x=w444, y=w446) -> (x*y=w443:dbl)
        "y dot 2" <- w443
        n178 = Multiply(x=w463, y=w418) -> (x*y=w424:dbl)
        n179 = Multiply(x=w460, y=w418) -> (x*y=w421:dbl)
        n180 = Multiply(x=w441, y=w418) -> (x*y=w419:dbl)
        "distance traveled 2" <- w419
        n181 = Multiply(x=w419, y=w442) -> (x*y=w440:dbl)
        "x traveled 2" <- w440
        n182 = Multiply(x=w419, y=w443) -> (x*y=w439:dbl)
        "y traveled 2" <- w439
        n183 = Add(x=w426, y=w440) -> (x+y=w438:dbl)
        n184 = Add(x=w427, y=w439) -> (x+y=w430:dbl)
        n185 = Multiply(x=w438, y=w418) -> (x*y=w422:dbl)
        n186 = Multiply(x=w418, y=w430) -> (x*y=w423:dbl)
        n187 = Divide(x=w438, y=9600.0) -> (x/y=w433:dbl)
        n188 = Divide(x=w430, y=9600.0) -> (x/y=w434:dbl)
        n189 = local read "start x"() -> (w431:dbl)
        n190 = local read "start y"() -> (w432:dbl)
        n191 = Add(x=w433, y=w431) -> (x+y=→"x position 2":dbl)
        n192 = Add(x=w434, y=w432) -> (x+y=→"y position 2":dbl)
      }
      n193 = while {
        tunnel: w204 -> [w510]
        stop <- FALSE stop-if-true
        # "left mid"
        n194 = xnode "Read/Write Control"("FPGA VI Reference In"=w510) -> ("ENC.A_a.CNTR"=→"ENC.A_a.CNTR":u32, "ENC.A_b.CNTR"=→"ENC.A_b.CNTR":u32, "ENC.A_c.CNTR"=→"ENC.A_c.CNTR":u32, "ENC.B_a.CNTR"=→"ENC.B_a.CNTR":u32, "ENC.B_b.CNTR"=→"ENC.B_b.CNTR":u32, "ENC.B_c.CNTR"=→"ENC.B_c.CNTR":u32)  [unwired: 1 in, 2 out]
        n195 = xnode "Read/Write Control"("FPGA VI Reference In"=w510) -> ("SYS.SELECTA"=→"SYS.SELECTA":u8)  [unwired: 1 in, 2 out]
        n196 = Wait (ms)(milliseconds to wait=u32 20) -> ()  [unwired: 1 out]
        n197 = case shown="True" "Encoder Reset" {
          tunnel: w510 -> [_ w521]
          frame False {
          }
          frame True {
            n198 = flat-sequence {
              tunnel: w521 -> [w526]
              tunnel: [w524] -> w523
              tunnel: w523 -> [w528]
              tunnel: [w528] -> w522
              tunnel: w522 -> [w531]
              tunnel: [w530] -> _
              frame #0 {
                w525 = u8 60 ("SYS.SELECTA")
                w527 = u8 3 ("ENC.B_c.CNFG")
                n199 = xnode "Read/Write Control"("FPGA VI Reference In"=w526, "ENC.A_a.CNFG"=w527, "ENC.A_b.CNFG"=w527, "ENC.A_c.CNFG"=w527, "ENC.B_a.CNFG"=w527, "ENC.B_b.CNFG"=w527, "ENC.B_c.CNFG"=w527, "SYS.SELECTA"=w525, "SYS.SELECTB"=w525) -> ("FPGA VI Reference Out"=w524:refnum<k20>)  [unwired: 1 in, 1 out]
              }
              frame #1 {
                n200 = Wait (ms)(milliseconds to wait=u32 10) -> ()  [unwired: 1 out]
              }
              frame #2 {
                w532 = u8 1 ("ENC.B_c.CNFG")
                n201 = xnode "Read/Write Control"("FPGA VI Reference In"=w531, "ENC.A_a.CNFG"=w532, "ENC.A_b.CNFG"=w532, "ENC.A_c.CNFG"=w532, "ENC.B_a.CNFG"=w532, "ENC.B_b.CNFG"=w532, "ENC.B_c.CNFG"=w532) -> ("FPGA VI Reference Out"=w530:refnum<k20>)  [unwired: 1 in, 1 out]
              }
            }
          }
        }
      }
      n202 = while {
        stop <- w292 stop-if-true
        n203 = case shown="2" "state" {
          tunnel: [_ _ _ _ w366] -> w292
          frame 0, Default {
            (unwired) TRUE
            # "state 0=start"
            n204 = flat-sequence {
              frame #0 {
                n205 = while {
                  stop <- w303 stop-if-true
                  n206 = Wait (ms)(milliseconds to wait=u32 500) -> ()  [unwired: 1 out]
                  n207 = local read "mining x 1"() -> (w308:dbl)
                  n208 = Not Equal?(x=w308, y=0.0) -> (x != y?=w304:bool)
                  n209 = And(x="position good?", y=w304) -> (x .and. y?=w303:bool)
                }
                n210 = local read "mining location"() -> (w296:dbl)
                n211 = case shown="1, Default" w296 {
                  tunnel: ["mining x 1" "mining x -1"] -> w293
                  tunnel: ["mining y 1" "mining y -1"] -> w295
                  tunnel: ["mining angle 1" "mining angle -1"] -> w294
                  frame 1, Default {
                  }
                  frame -1 {
                  }
                }
                "mining x" <- w293
                "mining y" <- w295
                "mining angle" <- w294
                n212 = local write "x goal"(w293) -> ()
              }
              frame #1 {
                n213 = local read "state"() -> (w310:dbl)
                n214 = local write "stop motors"(0.0 ("stop motors")) -> ()
                n215 = Add(x=w310, y=1.0) -> (x+y=w312:dbl)
                n216 = local write "state"(w312) -> ()
              }
              frame #2 {
                n217 = local read "state"() -> (w315:dbl)
                n218 = Equal?(x=w315, y=1.0) -> (x = y?=w313:bool)
                n219 = call "Display Message to User"("Enable"=w313) -> ()  [unwired: 9 in, 2 out]
              }
            }
          }
          frame 1 {
            # "state 1=forward"
            n220 = while {
              stop <- w316 stop-if-true
              (unwired) FALSE
              n221 = flat-sequence {
                tunnel: [w330] -> w316
                frame #0 {
                  n222 = local write "stop motors"(1.0) -> ()
                  "forward reverse" <- -1.0
                }
                frame #1 {
                  n223 = while {
                    stop <- w322 stop-if-true
                    n224 = call "Elapsed Time3"() -> ("Time has Elapsed"=w319:bool)  [unwired: 12 in, 7 out]
                    n225 = local read "x goal"() -> (w320:dbl)
                    n226 = case shown="True" w319 {
                      frame False {
                      }
                      frame True {
                        n227 = flat-sequence {
                          frame #0 {
                            n228 = local write "stop motors"(0.0) -> ()
                          }
                          frame #1 {
                            n229 = Wait (ms)(milliseconds to wait=u32 1000) -> ()  [unwired: 1 out]
                          }
                          frame #2 {
                            n230 = local write "stop motors"(1.0) -> ()
                          }
                        }
                      }
                    }
                    n231 = local read "loc_x"() -> (w321:dbl)
                    n232 = Greater Or Equal?(x=w321, y=w320) -> (x >= y?=w322:bool)
                  }
                }
                frame #2 {
                  n233 = local read "state"() -> (w326:dbl)
                  n234 = local write "stop motors"(0.0) -> ()
                  n235 = Add(x=w326, y=1.0) -> (x+y=w328:dbl)
                  n236 = local write "state"(w328) -> ()
                }
                frame #3 {
                  n237 = local read "state"() -> (w333:dbl)
                  n238 = Equal?(x=w333, y=2.0) -> (x = y?=w331:bool)
                  n239 = call "Display Message to User2"("Enable"=w331) -> ("OK"=w330:bool)  [unwired: 9 in, 1 out]
                }
              }
            }
          }
          frame 2 {
            # "state 2=dig"
            n240 = while {
              stop <- w334 stop-if-true
              (unwired) FALSE
              n241 = flat-sequence {
                tunnel: [w341] -> w334
                frame #0 {
                  n242 = while {
                    stop <- "digging complete?" stop-if-true
                  }
                }
                frame #1 {
                  n243 = shared-variable "RT myRIO Target - Overlord\\Localization_Variables_r0.lvlib\\loc_x"() -> (→"xstart_return":dbl)  [unwired: 1 in, 1 out]
                  n244 = local read "start x"() -> (w337:dbl)
                  n245 = local read "state"() -> (w339:dbl)
                  n246 = local write "x goal"(w337) -> ()
                  n247 = Add(x=w339, y=1.0) -> (x+y=w338:dbl)
                  n248 = local write "state"(w338) -> ()
                }
                frame #2 {
                  n249 = local read "state"() -> (w344:dbl)
                  n250 = Equal?(x=w344, y=3.0) -> (x = y?=w342:bool)
                  n251 = call "Display Message to User8"("Enable"=w342) -> ("OK"=w341:bool)  [unwired: 9 in, 1 out]
                }
              }
            }
          }
          frame 3 {
            # "state 3=return"
            n252 = while {
              stop <- w345 stop-if-true
              (unwired) FALSE
              # "dialog for testing and move to next case"
              # "measurement and control"
              # "chill and make sure loc is good"
              # "house keeping variables"
              n253 = flat-sequence {
                tunnel: [w362] -> w345
                frame #0 {
                  n254 = local read "start x"() -> (w347:dbl)
                  n255 = local write "stop motors"(1.0) -> ()
                  n256 = local read "right setpoint"() -> (w348:dbl)
                  n257 = local read "left setpoint"() -> (w349:dbl)
                  n258 = local write "forward reverse"(1.0) -> ()
                  n259 = local write "right setpoint"(w349) -> ()
                  n260 = local write "left setpoint"(w348) -> ()
                  n261 = local write "x goal"(w347) -> ()
                }
                frame #1 {
                  n262 = while {
                    stop <- w354 stop-if-true
                    n263 = local read "loc_x"() -> (w353:dbl)
                    n264 = call "Elapsed Time9"() -> ("Time has Elapsed"=w352:bool)  [unwired: 12 in, 7 out]
                    n265 = local read "x goal"() -> (w351:dbl)
                    n266 = case shown="True" w352 {
                      frame False {
                      }
                      frame True {
                        n267 = flat-sequence {
                          frame #0 {
                            n268 = local write "stop motors"(0.0) -> ()
                          }
                          frame #1 {
                            n269 = Wait (ms)(milliseconds to wait=u32 1000) -> ()  [unwired: 1 out]
                          }
                          frame #2 {
                            n270 = local write "stop motors"(1.0) -> ()
                          }
                        }
                      }
                    }
                    n271 = Greater Or Equal?(x=w353, y=w351) -> (x >= y?=w354:bool)
                  }
                }
                frame #2 {
                  n272 = local read "state"() -> (w359:dbl)
                  n273 = local write "stop motors"(0.0) -> ()
                  n274 = Add(x=w359, y=1.0) -> (x+y=w361:dbl)
                  n275 = local write "state"(w361) -> ()
                }
                frame #3 {
                  n276 = local read "state"() -> (w365:dbl)
                  n277 = Equal?(x=w365, y=4.0) -> (x = y?=w363:bool)
                  n278 = call "Display Message to User5"("Enable"=w363) -> ("OK"=w362:bool)  [unwired: 9 in, 1 out]
                }
              }
            }
          }
          frame 4 {
            (unwired) FALSE
            # "state 4=dump"
            n279 = flat-sequence {
              tunnel: [w372] -> w366
              frame #0 {
                n280 = while {
                  stop <- "dumping complete" stop-if-true
                }
              }
              frame #1 {
                n281 = local write "state"(1.0) -> ()
                n282 = local read "mining location"() -> (w370:dbl)
                n283 = Multiply(x=w370, y=-1.0) -> (x*y=w368:dbl)
                n284 = local write "mining location"(w368) -> ()
              }
              frame #2 {
                n285 = local read "state"() -> (w375:dbl)
                n286 = Equal?(x=w375, y=0.0) -> (x = y?=w373:bool)
                n287 = call "Display Message to User9"("Enable"=w373) -> ("OK"=w372:bool)  [unwired: 9 in, 1 out]
              }
            }
          }
        }
      }
      n288 = call "Tick Count"() -> ("Tick Count(uSec)"=w205:u32)
      n289 = while {
        shift-right: [w551] -> _
        shift-left: _ -> [w550]
        shift-right: [w548] -> _
        shift-left: w205 -> [w547]
        tunnel: w203 -> [w558]
        stop <- FALSE stop-if-true
        n290 = xnode "Read/Write Control"("FPGA VI Reference In"=w558) -> ("ENC.A_a.CNTR"=w557:u32, "ENC.A_b.CNTR"=w556:u32, "ENC.A_c.CNTR"=w555:u32, "ENC.B_a.CNTR"=w554:u32, "ENC.B_b.CNTR"=w553:u32, "ENC.B_c.CNTR"=w552:u32)  [unwired: 1 in, 2 out]
        n291 = call "Wait"("Count(mSec)"=u32 20) -> ()  [unwired: 1 out]
        n292 = Build Array(w557, w556, w555, w554, w553, w552) -> (w551:u32[])
        n293 = Subtract(x=w551, y=w550) -> (x-y=w549:u32[])
        n294 = call "Tick Count2"() -> ("Tick Count(uSec)"=w548:u32)
        n295 = Index Array(array=w549) -> (element #1=w546:u32, element #2=w545:u32, element #3=w544:u32, element #4=w543:u32, element #5=w542:u32, element #6=w541:u32)  [unwired: 6 in]
        n296 = Subtract(x=w548, y=w547) -> (x-y=w540:u32)
        n297 = call "Encoder-Velocity_Conversion (SubVI).vi"("delta  Encoder Count"=w546, "dt (uSec)"=w540) -> ("Rotational Velocity (RPS)"=w536:dbl)  [unwired: 7 in, 2 out]
        "LR Rot Velocity (rot/s)" <- w536
        n298 = call "Encoder-Velocity_Conversion (SubVI).vi"("delta  Encoder Count"=w541, "dt (uSec)"=w540) -> ("Rotational Velocity (RPS)"=w538:dbl)  [unwired: 7 in, 2 out]
        "RF Linear Velocity (rot/s)" <- w538
        n299 = call "Encoder-Velocity_Conversion (SubVI).vi"("delta  Encoder Count"=w545, "dt (uSec)"=w540) -> ("Rotational Velocity (RPS)"=w535:dbl)  [unwired: 7 in, 2 out]
        "LM Rot Velocity (rot/s)" <- w535
        n300 = call "Encoder-Velocity_Conversion (SubVI).vi"("delta  Encoder Count"=w544, "dt (uSec)"=w540) -> ("Rotational Velocity (RPS)"=w534:dbl)  [unwired: 7 in, 2 out]
        "LF Rot Velocity (rot/s)" <- w534
        n301 = call "Encoder-Velocity_Conversion (SubVI).vi"("delta  Encoder Count"=w543, "dt (uSec)"=w540) -> ("Rotational Velocity (RPS)"=w533:dbl)  [unwired: 7 in, 2 out]
        "RR Rot Velocity (rot/s)" <- w533
        n302 = call "Encoder-Velocity_Conversion (SubVI).vi"("delta  Encoder Count"=w542, "dt (uSec)"=w540) -> ("Rotational Velocity (RPS)"=w537:dbl)  [unwired: 7 in, 2 out]
        "RM Linear Velocity (rot/s)" <- w537
        n303 = Bundle("Rotational Velocity (RPS)"=w536, "Rotational Velocity (RPS)"=w535, "Rotational Velocity (RPS)"=w534, "Rotational Velocity (RPS)"=w533, "Rotational Velocity (RPS)"=w537, "Rotational Velocity (RPS)"=w538) -> (→"Current Rot Velocity (rot/s)":T4)  [unwired: 1 in]
      }
    }
  }
